vi "Exemple_Metrics_Adjusted_Rand_Score.vi"() -> ()   [LabVIEW 2020]
uses:
  Objet/3 - Model selection and evaluation/3.3 - Metrics and scoring/adjusted_rand_score/Adjusted_Rand_Score.vi
panel:
  out "error out":errorcluster caption="sortie d'erreur"
  out "Score":string
  in  "labels_pred":string[][](array[string])=[["0"], ["0"], ["1"], ["1"]]
  in  "labels_true":string[][](array[string])=[["0"], ["0"], ["1"], ["2"]]
  in  "error in":errorcluster caption="entrée d'erreur"
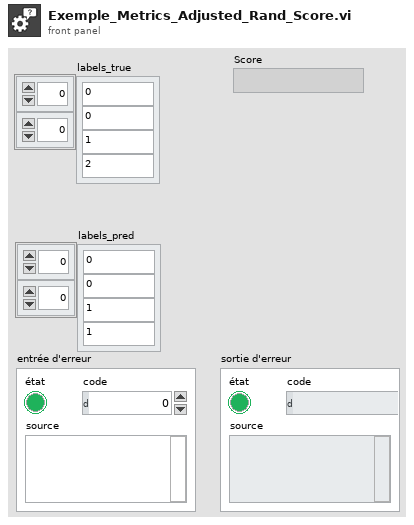
[diagram p1: front panel]
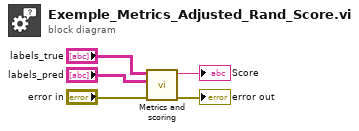
[diagram p0: block diagram]
diagram:
  n1 = call-poly "Metrics and scoring.vi"("error in"="error in", "labels_pred"="labels_pred", "labels_true"="labels_true") -> ("error out"=→"error out":errorcluster, "Score"=→"Score":string)  [unwired: 7 in]
